vi "Get Group Configuration.vi"(8 "error in (no error)":errorcluster, 11 "Component Configuration in":refnum<class "Core Component Configurations.lvclass">) -> (0 "error out":errorcluster, 1 "Tx Group Configuration":refnum<class "Configuration.lvclass">, 2 "Rx Group Configuration":refnum<class "Configuration.lvclass">, 3 "Component Configuration out":refnum<class "Core Component Configurations.lvclass">)   [LabVIEW 2017, in "DSF Core.lvlib" / "Core Component Configurations.lvclass"]
uses:
  Core Component Configurations.lvclass
  Configuration/Configuration.lvclass
  Configuration/Core/Group/Group Configuration.lvclass
  C:/Git/DSF/Core/Classes/Configuration/Configuration.lvclass
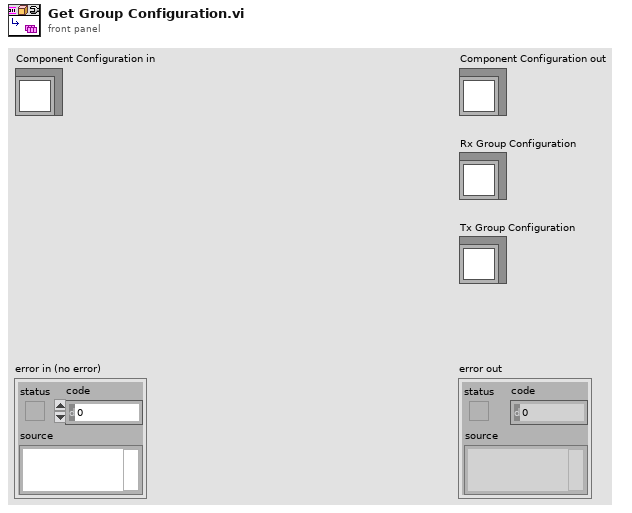
[diagram p1: front panel]
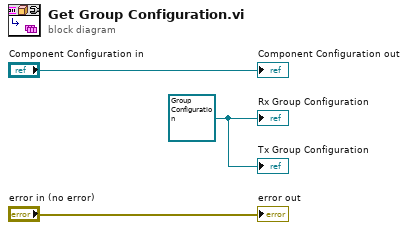
[diagram p0: block diagram]
diagram:
  w1 = refnum<class "Group Configuration.lvclass"> refnum ("DSF Core.lvlib:Group Configuration.lvclass")
  "error out" <- "error in (no error)"
  "Component Configuration out" <- "Component Configuration in"
  "Rx Group Configuration" <- w1
  "Tx Group Configuration" <- w1
